vi "SSL Log Sync.vi"(8 "error in (no error)":errorcluster, 10 "Slide":i64, 11 "Byte Stream File in":refnum<file>) -> (0 "error out":errorcluster, 2 "Offset":i64, 3 "Byte Stream File out":refnum<file>)   [LabVIEW 2017]
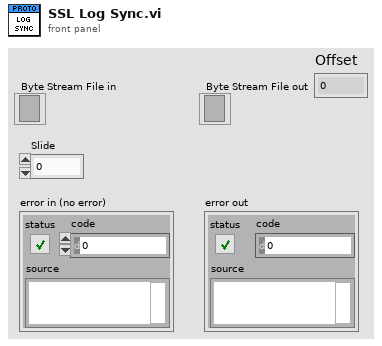
[diagram p1: front panel]
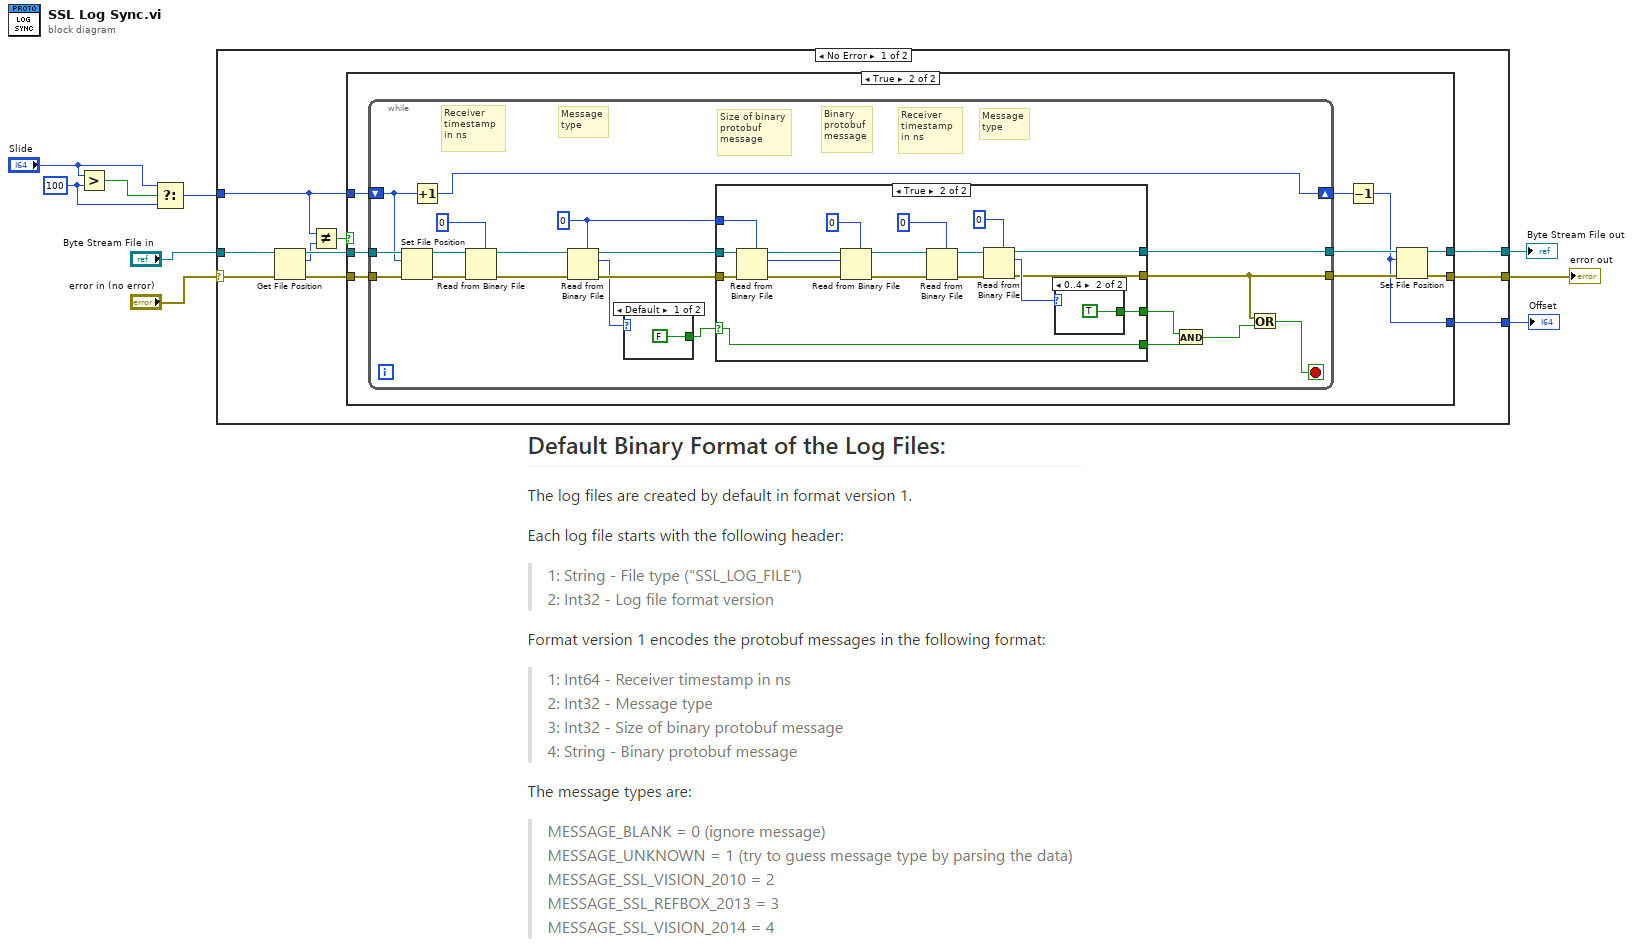
[diagram p0: block diagram]
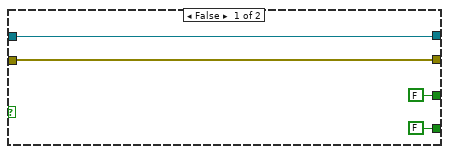
[diagram p3: hidden frame]
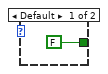
[diagram p4: hidden frame]
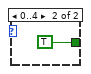
[diagram p5: hidden frame]
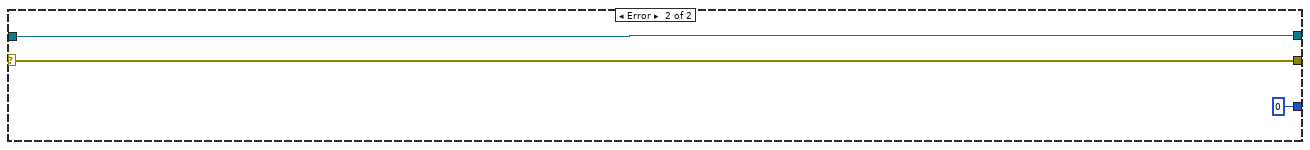
[diagram p6: hidden frame]
diagram:
  w1 = i64 100 ("y")
  n1 = Greater?(x="Slide", y=w1) -> (0:w3:bool)
  n2 = Select(t="Slide", s=w3, f=w1) -> (s? t:f=w4:i64)
  n3 = case shown="No Error" "error in (no error)" {
    selector: "error in (no error)" -> [w14 w79]
    tunnel: w4 -> [w12 _]
    tunnel: "Byte Stream File in" -> [w16 w80]
    tunnel: [w19 w79] -> w8
    tunnel: [w18 w80] -> w7
    tunnel: [w10 i64 0 ("Slide")] -> w5
    frame No Error {
      n4 = Get File Position(4:w14, 7:w16) -> (0:w17:errorcluster, 2:w11:i64, 3:w15:refnum<file>)
      n5 = Not Equal?(x=w12, y=w11) -> (x != y?=w13:bool)
      n6 = case shown="True" w13 {
        tunnel: w12 -> [w20 w31]
        tunnel: [w22 w28] -> w19
        tunnel: [w21 w27] -> w18
        tunnel: w17 -> [w22 w25]
        tunnel: w15 -> [w21 w24]
        tunnel: [w20 w23] -> w10
        frame False {
        }
        frame True {
          n7 = while {
            tunnel: w24 -> [w51]
            tunnel: w25 -> [w50]
            shift-right: [w41] -> w26
            shift-left: w31 -> [w42]
            tunnel: [w37] -> w30
            tunnel: [w35] -> w29
            stop <- w34 stop-if-true
            w45 = 0 ("data type")
            # "Receiver \ntimestamp \nin ns"
            # "Message\ntype"
            # "Binary\nprotobuf\nmessage"
            # "Size of binary\nprotobuf \nmessage"
            # "Receiver \ntimestamp \nin ns"
            # "Message\ntype"
            n8 = Set File Position(offset (in bytes) (0)=w42, refnum=w51, error in=w50) -> (refnum out=w43:refnum<file>, error out=w44:errorcluster)  [unwired: 1 in]
            n9 = Increment(x=w42) -> (x+1=w41:i64)
            n10 = Read from Binary File(5:i64 0 ("data type"), 8:w44, 11:w43) -> (0:w48:errorcluster, 3:w49:refnum<file>)  [unwired: 3 in, 2 out]
            n11 = Read from Binary File(5:w45, 8:w48, 11:w49) -> (0:w46:errorcluster, 2:w39:i32, 3:w47:refnum<file>)  [unwired: 3 in, 1 out]
            n12 = case shown="Default" w39 {
              tunnel: [FALSE TRUE] -> w33
              frame Default {
              }
              frame 0..4 {
              }
            }
            n13 = case shown="True" w33 {
              selector: w33 -> [_ w56]
              tunnel: w47 -> [w52 w72]
              tunnel: w46 -> [w53 w70]
              tunnel: w45 -> [_ w68]
              tunnel: [FALSE w59] -> w38
              tunnel: [w52 w58] -> w37
              tunnel: [w53 w57] -> w35
              tunnel: [FALSE w56] -> w32
              frame False {
              }
              frame True {
                n14 = Read from Binary File(5:w68, 8:w70, 11:w72) -> (0:w69:errorcluster, 2:w67:i32, 3:w71:refnum<file>)  [unwired: 3 in, 1 out]
                n15 = Read from Binary File(5:u8 0 ("data type"), 8:w69, 10:w67, 11:w71) -> (0:w64:errorcluster, 3:w65:refnum<file>)  [unwired: 2 in, 2 out]
                n16 = Read from Binary File(5:i64 0 ("data type"), 8:w64, 11:w65) -> (0:w62:errorcluster, 3:w61:refnum<file>)  [unwired: 3 in, 2 out]
                n17 = Read from Binary File(5:0 ("data type"), 8:w62, 11:w61) -> (0:w57:errorcluster, 2:w60:i32, 3:w58:refnum<file>)  [unwired: 3 in, 1 out]
                n18 = case shown="0..4" w60 {
                  tunnel: [FALSE TRUE] -> w59
                  frame Default {
                  }
                  frame 0..4 {
                  }
                }
              }
            }
            n19 = And(x=w38, y=w32) -> (x .and. y?=w36:bool)
            n20 = Or(x=w35, y=w36) -> (x .or. y?=w34:bool)
          }
          n21 = Decrement(x=w26) -> (x-1=w23:i64)
          n22 = Set File Position(offset (in bytes) (0)=w23, refnum=w30, error in=w29) -> (refnum out=w27:refnum<file>, error out=w28:errorcluster)  [unwired: 1 in]
        }
      }
    }
    frame Error {
    }
  }
  "Byte Stream File out" <- w7
  "error out" <- w8
  "Offset" <- w5
